vi "SLSC Get Capabilities NVMEM String.vi"(8 "error in (no error)":errorcluster, 11 "SLSC Device":refnum<k21>) -> (0 "error out":errorcluster, 3 "capabilities NVMEM":string)   [LabVIEW 2017, in "SLSC EDS API.lvlib"]
doc: "Reads the capabilities NVMEM section for an SLSC module."
uses:
  SLSC EDS API.lvlib
  <vilib>/SLSC/Initialize Session with NVMEM Areas.vi
  <vilib>/SLSC/Close Session.vi
  <vilib>/SLSC/SLSC.lvlib
  <resource>/objmgr/slsc.rc
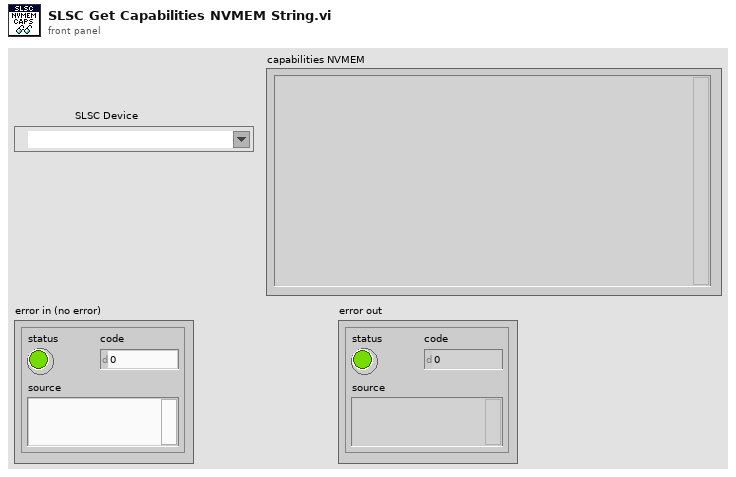
[diagram p1: front panel]
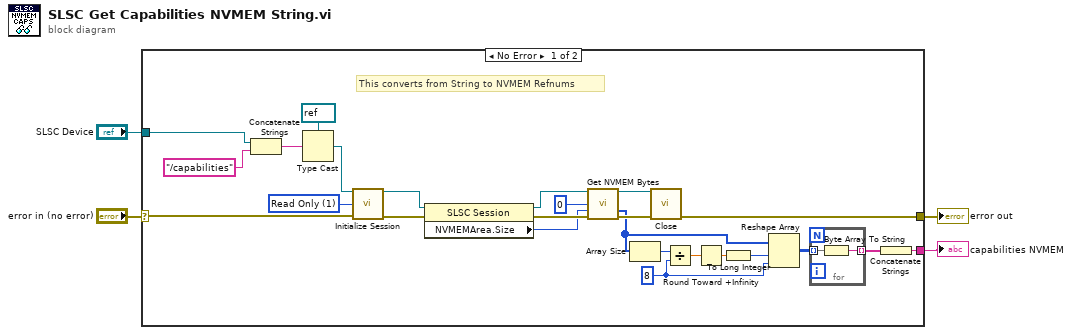
[diagram p0: block diagram]
diagram:
  n1 = case shown="No Error" "error in (no error)" {
    selector: "error in (no error)" -> [w6 w32]
    tunnel: [w8 w32] -> w4
    tunnel: [w7 _] -> w2
    tunnel: "SLSC Device" -> [w5 _]
    frame No Error {
      w18 = 8 ("dimension size")
      w21 = 1 items=["None"=0, "Read Only"=1, "Read/Write"=3] ("reservation access (Read/Write)")
      # "This converts from String to NVMEM Refnums"
      n2 = Concatenate Strings(w5, "/capabilities" ("string")) -> (w11:string)
      n3 = Type Cast(type=refnum<k21> refnum ("NVMEM area"), x=w11) -> (*(type *) &x=w10:refnum<k21>)
      n4 = call-poly <vilib>:"Initialize Session.vi"("NVMEM areas"=w10, "reservation access (Read/Write)"=w21, "error in (no error)"=w6) -> ("session out"=w23:refnum<k21>, "error out"=w22:errorcluster)  [unwired: 11 in]
      n5 = property class="SLSC Session"(reference=w23, error in=w22) -> (reference out=w26:refnum<k21>, error out=w25:errorcluster, "NVMEMArea.Size"=w24:u32)
      n6 = call <vilib>:"Get NVMEM Bytes.vi"("session in"=w26, "data address"=u32 0, "data size"=w24, "error in (no error)"=w25) -> ("session out"=w29:refnum<k21>, "data out"=w14:u8[], "error out"=w28:errorcluster)  [unwired: 7 in, 2 out]
      n7 = Array Size(array=w14) -> (size(s)=w19:i32)
      n8 = call-poly <vilib>:"Close.vi"("session in"=w29, "error in (no error)"=w28) -> ("error out"=w8:errorcluster)  [unwired: 13 in]
      n9 = Divide(x=w19, y=w18) -> (x/y=w17:dbl)
      n10 = Round Toward +Infinity(x=w17) -> (ceil(x): smallest int >= x=w16:dbl)
      n11 = To Long Integer(number=w16) -> (32bit integer=w15:i32)
      n12 = Reshape Array(w14, w15, w18) -> (w13:u8[][])
      n13 = for {
        tunnel: w13 -> [w31] mode=indexing
        tunnel: [w30] -> w9 mode=indexing
        n14 = Byte Array To String(unsigned byte array=w31) -> (string=w30:string)
      }
      n15 = Concatenate Strings(w9) -> (w7:string)
    }
    frame Error {
    }
  }
  "error out" <- w4
  "capabilities NVMEM" <- w2
